vi "Save Pulse Data.vi"(8 "error in (no error)":errorcluster, 11 "RP I-V Driver in":refnum<class "RP I-V Driver.lvclass">) -> (0 "error out":errorcluster, 3 "RP I-V Driver out":refnum<class "RP I-V Driver.lvclass">)   [LabVIEW 2024, in "RP I-V Driver.lvclass"]
uses:
  RP I-V Driver.lvclass
  Instruments/Pulse Driver/Pulse Driver.lvclass/Pulse Driver.ctl
  Red Pitaya Digitizer/Red Pitaya Digitizer.lvclass/Red Pitaya Digitizer.ctl
  Instruments/Pulse Driver/Read tdms file.vi
  Red Pitaya Digitizer/Read Logic tag.vi
  Instruments/Pulse Driver/Write tdms file.vi
  RP Instrument/RP Instrument.lvclass
  RP I-V Driver.lvclass/RP I-V Driver.ctl
panel:
  out "max value":i32
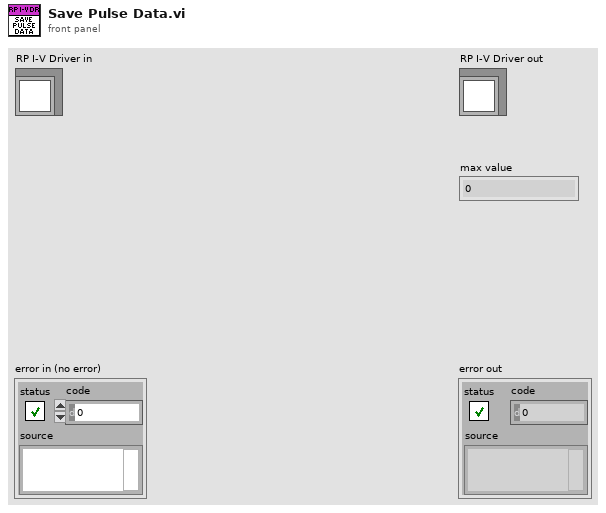
[diagram p1: front panel]
types:
  T1 = enum16{"big-endian, network order", "native, host order", "little-endian"}
  T2 = typedef "RP I-V Configuration.ctl" = cluster{"I-V parameters":T3, "Ranges":dbl[], "Post-trigger delay":dbl, "Post-trigger duration":dbl, "Output delay":dbl}
  T3 = typedef "I-V parameters.ctl" = cluster{"Start magnitude":dbl, "Magnitude increment":dbl, "End magnitude":dbl, "Ramp length":i32, "Top  length":i32, "Threshold ":dbl, "Processing delay":u16, "Output gain ":dbl, "Interpolation":i32, "Stop after":u16, "Detector window":i32}
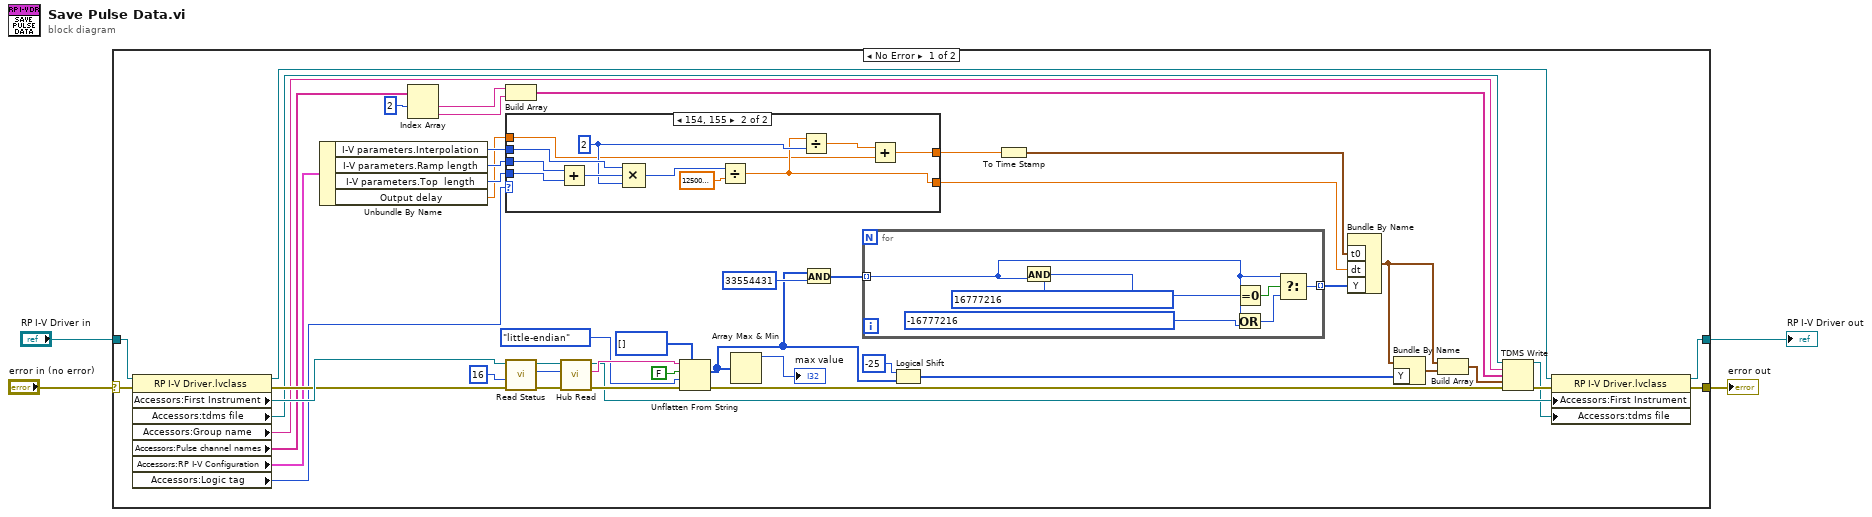
[diagram p0: block diagram]
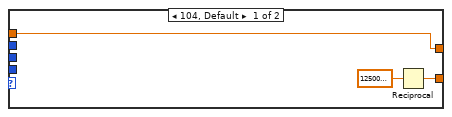
[diagram p2: hidden frame]
diagram:
  n1 = case shown="No Error" "error in (no error)" {
    selector: "error in (no error)" -> [w50 w73]
    tunnel: [w21 w73] -> w3
    tunnel: [w19 w72] -> w1
    tunnel: "RP I-V Driver in" -> [w49 w72]
    frame No Error {
      n2 = property class="RP I-V Driver.lvclass"(reference=w49, error in=w50) -> (reference out=w20:refnum<class "RP I-V Driver.lvclass">, error out=w47:errorcluster, "Accessors:First Instrument"=w48:refnum<class "RP Instrument.lvclass">, "Accessors:tdms file"=w37:refnum<k34>, "Accessors:Group name"=w36:string, "Accessors:Pulse channel names"=w34:string[], "Accessors:RP I-V Configuration"=w31:T2, "Accessors:Logic tag"=w30:u16)
      n3 = Unbundle By Name(w31) -> ("I-V parameters.Interpolation"=w29:i32, "I-V parameters.Ramp length"=w28:i32, "I-V parameters.Top  length"=w27:i32, "Output delay"=w25:dbl)
      n4 = Index Array(array=w34, index #1=2 ("index")) -> (element #1=w32:string, element #2=w13:string)  [unwired: 1 in]
      n5 = Build Array(w32, w13) -> (w14:string[])
      n6 = case shown="154, 155" w30 {
        tunnel: [w59 w64] -> w26
        tunnel: w29 -> [_ w68]
        tunnel: w28 -> [_ w71]
        tunnel: w27 -> [_ w70]
        tunnel: w25 -> [w58 w62]
        tunnel: [w58 w61] -> w24
        frame 104, Default {
          n7 = Reciprocal(x=125000000.0 ("y")) -> (1/x=w59:dbl)
        }
        frame 154, 155 {
          w65 = 2 ("value")
          n8 = Add(x=w71, y=w70) -> (x+y=w69:i32)
          n9 = Compound Arithmetic op=MULTIPLY(w68, w69, w65) -> (w67:i32)
          n10 = Divide(x=w67, y=125000000.0) -> (x/y=w64:dbl)
          n11 = Divide(x=w64, y=w65) -> (x/y=w63:dbl)
          n12 = Add(x=w63, y=w62) -> (x+y=w61:dbl)
        }
      }
      n13 = call-dynamic "Read Status.vi"("error in (no error)"=w47, "Status offset"=u64 16, "RP Instrument in"=w48) -> ("error out"=w43:errorcluster, "Status response"=w44:u32, "RP Instrument out"=w45:refnum<class "RP Instrument.lvclass">)  [unwired: 6 in]
      n14 = call-dynamic "Hub Read.vi"("error in (no error)"=w43, "Number of samples"=w44, "RP Instrument in"=w45) -> ("error out"=w42:errorcluster, "data out"=w41:string, "RP Instrument out"=w18:refnum<class "RP Instrument.lvclass">)  [unwired: 6 in]
      n15 = Unflatten From String(type=i32[] [], binary string=w41, data includes array or string size? (T)=FALSE, byte order (0:big-endian, network order)=T1."little-endian", error in (no error)=w42) -> (value=w9:i32[], error out=w35:errorcluster)  [unwired: 1 out]
      n16 = Array Max & Min(array=w9) -> (max value=→"max value":i32)  [unwired: 3 out]
      n17 = And(x=w9, y=33554431) -> (x .and. y?=w6:i32[])
      n18 = for {
        tunnel: w6 -> [w51] mode=indexing
        tunnel: [w52] -> w5 mode=indexing
        n19 = And(x=16777216, y=w51) -> (x .and. y?=w56:i32)
        n20 = Equal To 0?(x=w56) -> (x = 0?=w55:bool)
        n21 = Or(x=w51, y=-16777216) -> (x .or. y?=w53:i32)
        n22 = Select(t=w51, s=w55, f=w53) -> (s? t:f=w52:i32)
      }
      n23 = Logical Shift(y=i16 -25, x=w9) -> (x << y=w7:i32[])
      n24 = To Time Stamp(1:w24) -> (0:w23:timestamp)
      n25 = Bundle By Name("t0"=w23, "dt"=w26, "Y"=w5) -> (w11:waveform(i32))  [unwired: 1 in]
      n26 = Bundle By Name(cluster=w11, "Y"=w7) -> (w10:waveform(i32))
      n27 = Build Array(w11, w10) -> (w12:waveform(i32)[])
      n28 = TDMS Write(0:w37, 5:w36, 7:w14, 9:w12, 11:w35) -> (4:w15:refnum<k34>, 15:w22:errorcluster)  [unwired: 1 in, 2 out]
      n29 = property class="RP I-V Driver.lvclass"(reference=w20, error in=w22, "Accessors:First Instrument"=w18, "Accessors:tdms file"=w15) -> (reference out=w19:refnum<class "RP I-V Driver.lvclass">, error out=w21:errorcluster)
    }
    frame Error {
    }
  }
  "error out" <- w3
  "RP I-V Driver out" <- w1
